vi "Convert Single Frame (CAN to Raw).vi"(8 "error in":errorcluster, 11 "CAN frame":T1 {"payload" format="%x"; "timestamp" format="%<%.7X\n%x>T"; "type" items=["CAN Data"=0, "CAN Remote"=1, "CAN Bus Error"=2, "CAN 2.0 Data"=8, "CAN FD Data"=16, "CAN FD+BRS Data"=24, "J1939 Data"=192, "Delay"=224, "Log Trigger"=225, "Start Trigger"=226]; "identifier" format="%x"}) -> (0 "error out":errorcluster, 3 "Raw U32":u32[](array[numeric]))   [LabVIEW 2020, in "985x Support Addon Engine.lvlib"]
doc: "Convert a single CAN frame to insert into array of raw frame data."
uses:
  985x Support Addon Engine.lvlib
  <vilib>/xnet/xnet.llb/XNET Frame CAN.ctl
  <vilib>/xnet/xnet.llb/XNET Frame Type CAN.ctl
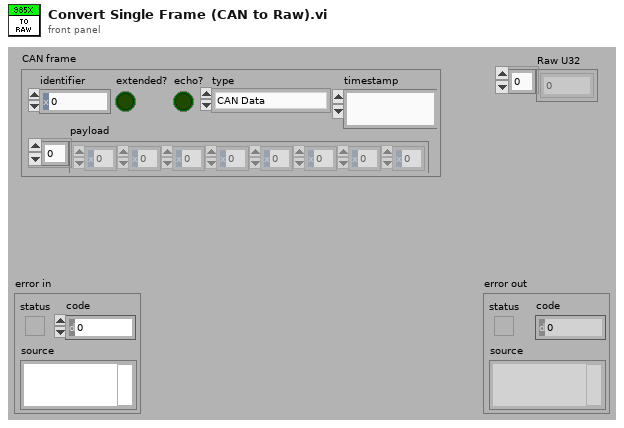
[diagram p1: front panel]
types:
  T1 = typedef "XNET Frame CAN.ctl" = cluster{"timestamp":timestamp, "payload":u8[], "identifier":u32, "type":T2, "extended?":bool, "echo?":bool}
  T2 = typedef "XNET Frame Type CAN.ctl" = u8
  T3 = enum16{"big-endian, network order", "native, host order", "little-endian"}
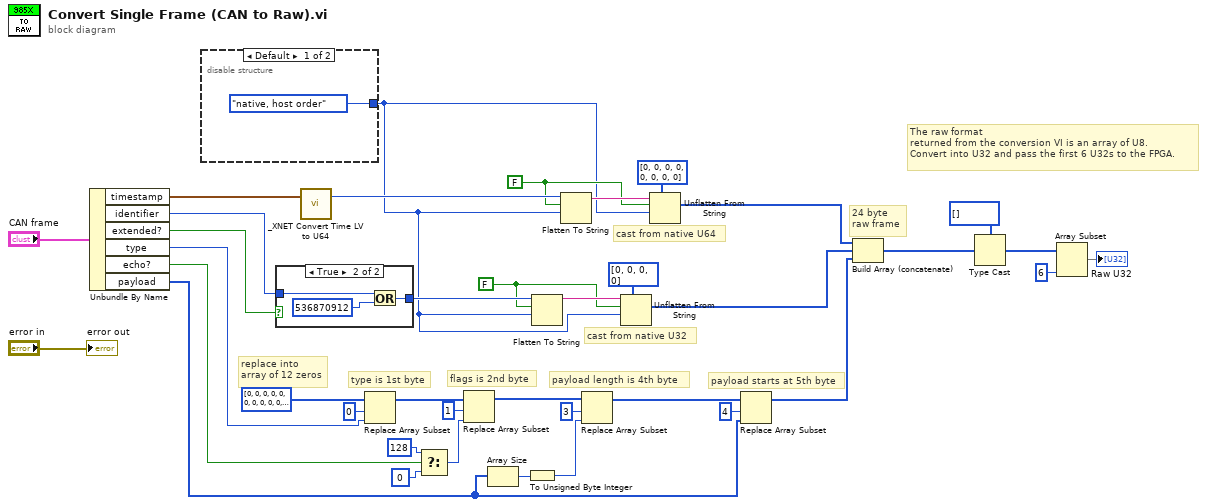
[diagram p0: block diagram]
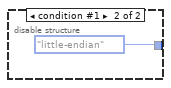
[diagram p2: hidden frame]
diagram:
  w16 = FALSE ("prepend array or string size? (T)")
  w15 = FALSE ("prepend array or string size? (T)")
  # "The raw format\nreturned from the conversion VI is an array of U8.\nConvert into U32 and pass the first 6 U32s to the FPGA."
  # "flags is 2nd byte"
  # "24 byte\nraw frame"
  # "payload starts at 5th byte"
  # "payload length is 4th byte"
  # "type is 1st byte"
  # "replace into\narray of 12 zeros"
  # "cast from native U32"
  # "cast from native U64"
  n1 = Unbundle By Name("CAN frame") -> ("timestamp"=w34:timestamp, "identifier"=w36:u32, "extended?"=w35:bool, "type"=w22:T2, "echo?"=w7:bool, "payload"=w11:u8[])
  n2 = disable-structure shown="Default" {
    disable-tunnel: [T3."native, host order" ("byte order (0:big-endian, network order)") T3."little-endian" ("byte order (0:big-endian, network order)")] -> w1
    frame condition #0 (active) {
    }
    frame condition #1 {
    }
  }
  n3 = case shown="True" w35 {
    tunnel: w36 -> [w41 w43]
    tunnel: [w41 w42] -> w26
    frame False {
    }
    frame True {
      n4 = Or(x=w43, y=u32 536870912) -> (x .or. y?=w42:u32)
    }
  }
  n5 = call <vilib>:"_XNET Convert Time LV to U64.vi"("Time LV"=w34) -> ("Time U64"=w31:u64)  [unwired: 2 out]
  n6 = Replace Array Subset(array=u8[] [0, 0, 0, 0, 0, 0, 0, 0, 0, 0, 0, 0], new element=w22, index=0) -> (w13:u8[])
  n7 = Select(t=u8 128 ("index"), s=w7, f=u8 0 ("index")) -> (s? t:f=w10:u8)
  n8 = Replace Array Subset(array=w13, new element=w10, index=1) -> (w12:u8[])
  n9 = Array Size(array=w11) -> (size(s)=w33:i32)
  n10 = To Unsigned Byte Integer(number=w33) -> (unsigned 8bit integer=w20:u8)
  n11 = Flatten To String(anything=w26, prepend array or string size? (T)=w16, byte order (0:big-endian, network order)=w1) -> (data string=w28:string)  [unwired: 1 in, 2 out]
  n12 = Flatten To String(anything=w31, prepend array or string size? (T)=w15, byte order (0:big-endian, network order)=w1) -> (data string=w32:string)  [unwired: 1 in, 2 out]
  n13 = Replace Array Subset(array=w12, new element=w20, index=3) -> (w18:u8[])
  n14 = Unflatten From String(type=u8[] [0, 0, 0, 0], binary string=w28, data includes array or string size? (T)=w16, byte order (0:big-endian, network order)=w1) -> (value=w25:u8[])  [unwired: 1 in, 2 out]
  n15 = Unflatten From String(type=u8[] [0, 0, 0, 0, 0, 0, 0, 0], binary string=w32, data includes array or string size? (T)=w15, byte order (0:big-endian, network order)=w1) -> (value=w29:u8[])  [unwired: 1 in, 2 out]
  n16 = Replace Array Subset(array=w18, new element=w11, index=4) -> (w17:u8[])
  n17 = Build Array (concatenate)(w29, w25, w17) -> (w4:u8[])
  n18 = Type Cast(type=u32[] [], x=w4) -> (*(type *) &x=w2:u32[])
  n19 = Array Subset(array=w2, length=6) -> (→"Raw U32":u32[])  [unwired: 1 in]
  "error out" <- "error in"
